vi "Material-Glue-Tree-AddItems.vi"(0 "Tree Ctl Ref":refnum<vi>, 5 "Tree Items to Create":T1[](array[typedef]), 7 "Delete Tree Items First?":bool=TRUE, 9 "Collapse all new items?":bool=TRUE, 11 "error in":errorcluster) -> (4 "Tree Ctl Ref out":refnum<vi>, 6 "Tree Item Tags Created":string[](array[string]), 15 "error out":errorcluster)   [LabVIEW 2013]
uses:
  Material-Glue-TreeItem.ctl
  Reuse Library/featherweight/Core/Collection/FTW-Collection.lvclass
panel:
  # "Inputs"
  # "Outputs"
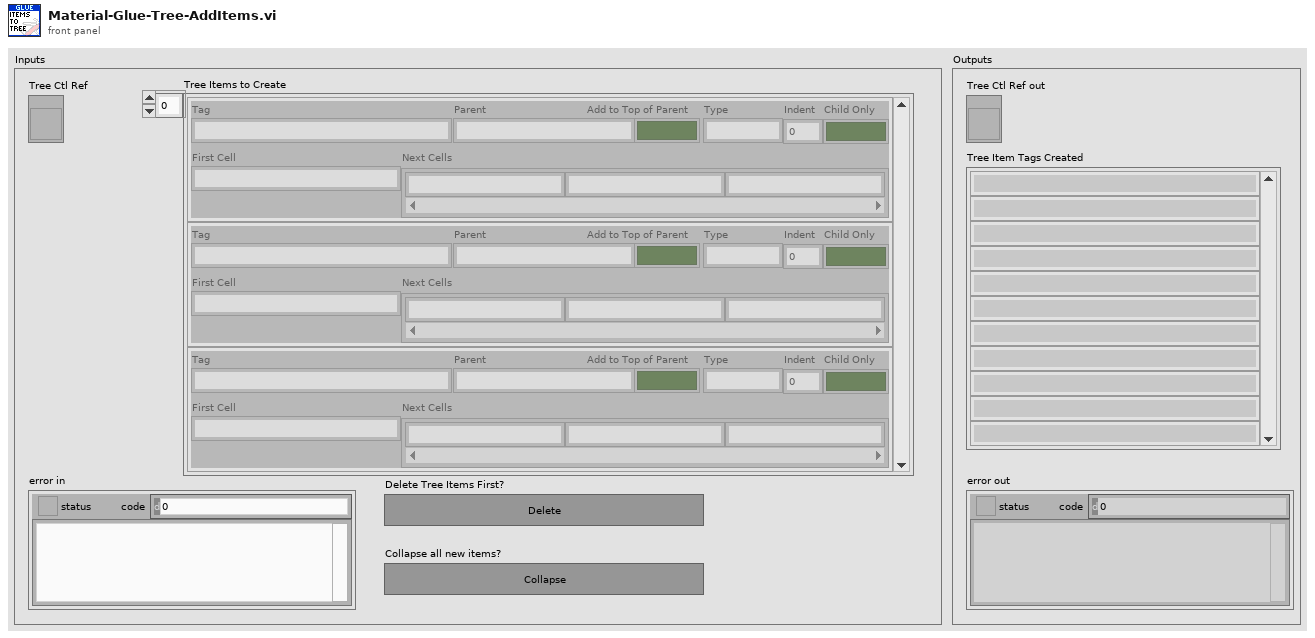
[diagram p1: front panel]
types:
  T1 = typedef "Material-Glue-TreeItem.ctl" = cluster{"Tag":string, "Parent":string, "Add to Top of Parent":bool, "Type":string, "Indent":i32, "Child Only":bool, "First Cell":string, "Next Cells":string[]}
  T2 = cluster{"Left Cell String":string, "Child Text":string[], "Child Tag":string, "Item Indent":i32, "Child Only?":bool, "Glyph Index":i32}
  T3 = cluster{"Position":i32, "Tag":string, "Parent":string}
  T4 = typedef "FTW-Collection-KeyValuePair.ctl" = cluster{"Key":string, "Value":string}
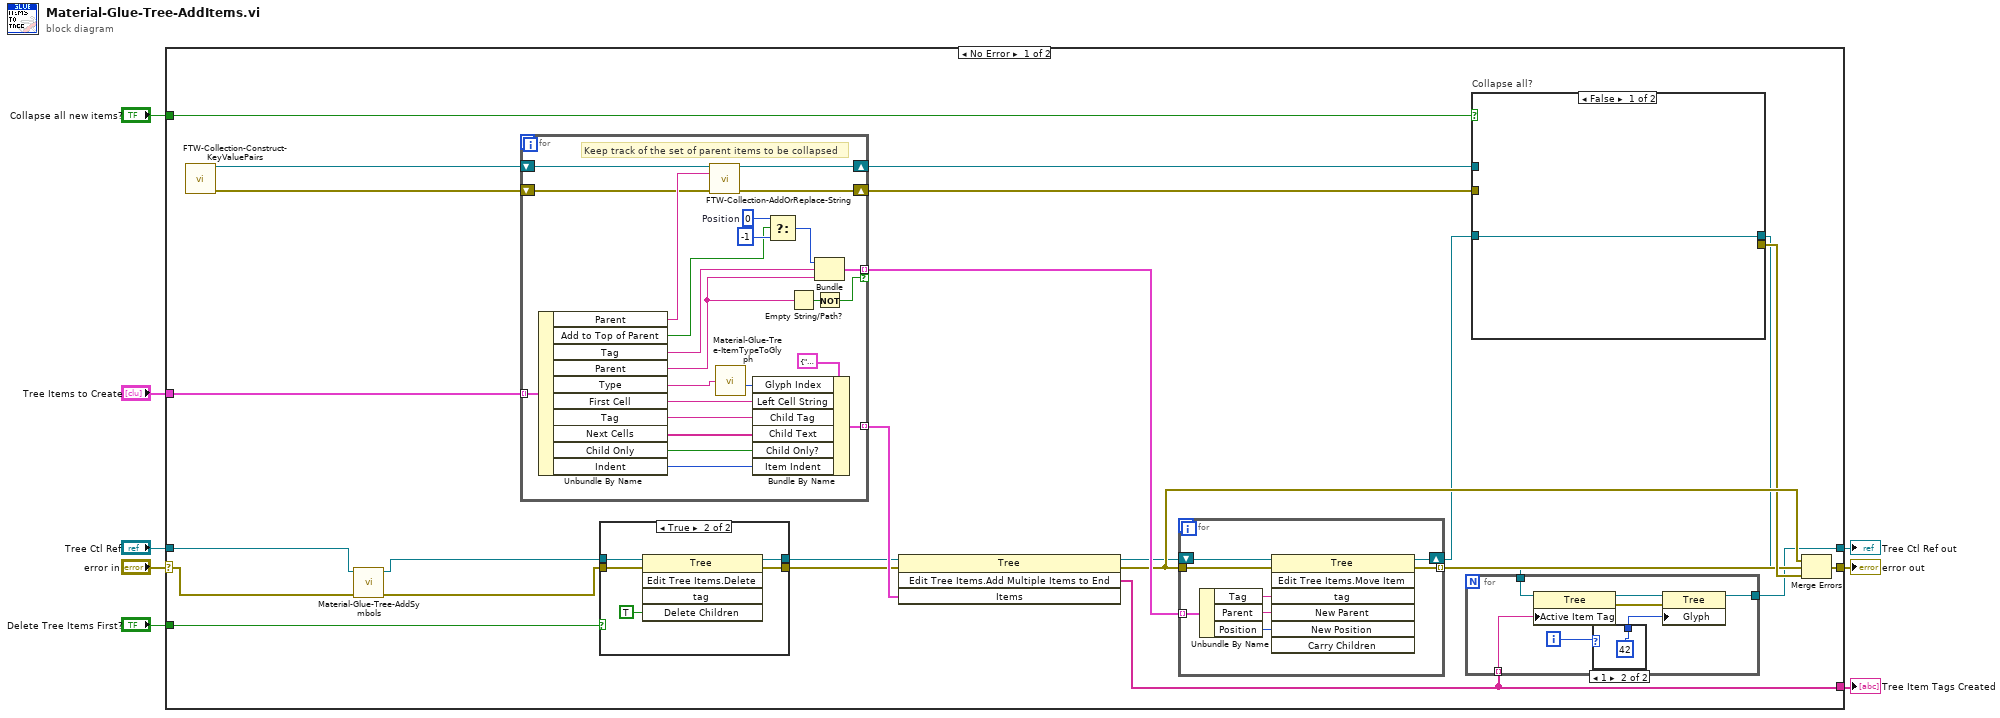
[diagram p0: block diagram]
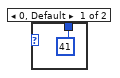
[diagram p2: hidden frame]
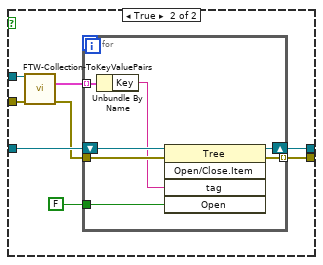
[diagram p3: hidden frame]
diagram:
  n1 = case shown="No Error" "error in" {
    selector: "error in" -> [w12 w98]
    tunnel: [w29 w98] -> w8
    tunnel: "Tree Ctl Ref" -> [w15 w97]
    tunnel: "Tree Items to Create" -> [w30 _]
    tunnel: "Delete Tree Items First?" -> [w24 _]
    tunnel: "Collapse all new items?" -> [w20 _]
    tunnel: [w9 w97] -> w2
    tunnel: [w11 _] -> w1
    frame No Error {
      n2 = call "FTW-Collection-Construct-KeyValuePairs.vi"() -> ("Collection"=w18:refnum<class "FTW-Collection.lvclass">, "error out"=w17:errorcluster)  [unwired: 14 in]
      n3 = call "Material-Glue-Tree-AddSymbols.vi"("error in (no error)"=w12, "TreeControl in"=w15) -> ("error out"=w13:errorcluster, "TreeControl out"=w14:refnum<vi>)  [unwired: 8 in]
      n4 = for {
        tunnel: [w87] -> w32 mode=indexing
        tunnel: w30 -> [w88] mode=indexing
        tunnel: [w65] -> w31 mode=indexing if=w75
        shift-right: [w67] -> w23
        shift-left: w18 -> [w69]
        shift-right: [w66] -> w22
        shift-left: w17 -> [w68]
        w77 = 0  # Position
        # "Keep track of the set of parent items to be collapsed"
        n5 = Unbundle By Name(w88) -> ("Parent"=w70:string, "Add to Top of Parent"=w74:bool, "Tag"=w71:string, "Parent"=w72:string, "Type"=w86:string, "First Cell"=w85:string, "Tag"=w83:string, "Next Cells"=w82:string[], "Child Only"=w81:bool, "Indent"=w80:i32)
        n6 = call "FTW-Collection-AddOrReplace-String.vi"("Collection"=w69, "Key"=w70, "error in"=w68) -> ("Collection out"=w67:refnum<class "FTW-Collection.lvclass">, "error out"=w66:errorcluster)  [unwired: 10 in, 1 out]
        n7 = call "Material-Glue-Tree-ItemTypeToGlyph.vi"("Item Type"=w86) -> ("Glyph Index"=w84:i32)  [unwired: 1 in, 2 out]
        n8 = Bundle By Name(cluster=T2 {"Left Cell String"="", "Child Text"=[], "Child Tag"="", "Item Indent"=0, "Child Only?"=FALSE, "Glyph Index"=0} ("Item"), "Glyph Index"=w84, "Left Cell String"=w85, "Child Tag"=w83, "Child Text"=w82, "Child Only?"=w81, "Item Indent"=w80) -> (w87:T2)
        n9 = Select(t=w77, s=w74, f=-1) -> (s? t:f=w73:i32)
        n10 = Empty String/Path?(string/path=w72) -> (empty?=w79:bool)
        n11 = Bundle("Position"=w73, "Tag"=w71, "Parent"=w72) -> (w65:T3)  [unwired: 1 in]
        n12 = Not(x=w79) -> (.not. x?=w75:bool)
      }
      n13 = case shown="True" w24 {
        tunnel: w14 -> [w59 w63]
        tunnel: [w59 w62] -> w26
        tunnel: w13 -> [w58 w61]
        tunnel: [w58 w60] -> w25
        frame False {
        }
        frame True {
          n14 = invoke on="Invoke Node" class="Tree" method="Edit Tree Items.Delete"(reference=w63, error in=w61, "Delete Children"=TRUE ("Delete Children?")) -> (reference out=w62:refnum<vi>, error out=w60:errorcluster)  [unwired: 2 in, 3 out]
        }
      }
      n15 = invoke on="Invoke Node" class="Tree" method="Edit Tree Items.Add Multiple Items to End"(reference=w26, error in=w25, "Items"=w32) -> (reference out=w27:refnum<vi>, error out=w28:errorcluster, "Edit Tree Items:Add Multiple Items to End"=w11:string[])  [unwired: 1 in, 1 out]
      n16 = for {
        tunnel: w28 -> [w96]
        tunnel: [w95] -> w16 mode=indexing
        tunnel: w31 -> [w93] mode=indexing
        shift-right: [w89] -> w21
        shift-left: w27 -> [w94]
        n17 = Unbundle By Name(w93) -> ("Tag"=w92:string, "Parent"=w91:string, "Position"=w90:i32)
        n18 = invoke on="Invoke Node" class="Tree" method="Edit Tree Items.Move Item"(reference=w94, error in=w96, "tag"=w92, "New Parent"=w91, "New Position"=w90) -> (reference out=w89:refnum<vi>, error out=w95:errorcluster)  [unwired: 2 in, 5 out]
      }
      n19 = case "Collapse all?" shown="False" w20 {
        tunnel: w23 -> [_ w46]
        tunnel: w22 -> [_ w45]
        tunnel: w21 -> [w42 w50]
        tunnel: [_ w49] -> w19
        tunnel: [w42 w48] -> w10
        frame False {
        }
        frame True {
          n20 = call "FTW-Collection-ToKeyValuePairs.vi"("Collection"=w46, "error in"=w45) -> ("Key-Value Pairs"=w43:T4[], "error out"=w44:errorcluster)  [unwired: 11 in, 1 out]
          n21 = for {
            tunnel: [w57] -> w49 mode=indexing
            tunnel: w43 -> [w52] mode=indexing
            tunnel: w44 -> [w55]
            shift-right: [w54] -> w48
            shift-left: w50 -> [w56]
            tunnel: FALSE ("Open?") -> [w53]
            n22 = Unbundle By Name(w52) -> ("Key"=w51:string)
            n23 = invoke on="Invoke Node" class="Tree" method="Open/Close.Item"(reference=w56, error in=w55, "tag"=w51, "Open"=w53) -> (reference out=w54:refnum<vi>, error out=w57:errorcluster)  [unwired: 1 in, 3 out]
          }
        }
      }
      n24 = for {
        tunnel: w11 -> [w36] mode=indexing
        tunnel: w10 -> [w35]
        tunnel: [w34] -> w9
        i -> [w33]
        n25 = property class="Tree"(reference=w35, "Active Item Tag"=w36) -> (reference out=w39:refnum<vi>, error out=w38:errorcluster)  [unwired: 1 in]
        n26 = case shown="1" w33 {
          tunnel: [41 ("Active Item:Symbol Index") 42 ("Active Item:Symbol Index")] -> w37
          frame 0, Default {
          }
          frame 1 {
          }
        }
        n27 = property class="Tree"(reference=w39, error in=w38, "Glyph"=w37) -> (reference out=w34:refnum<vi>)  [unwired: 1 out]
      }
      n28 = Merge Errors(w28, w16, w19) -> (w29:errorcluster)
    }
    frame Error {
    }
  }
  "error out" <- w8
  "Tree Ctl Ref out" <- w2
  "Tree Item Tags Created" <- w1
